vi "loopmod.vi"() -> ()   [LabVIEW 2018, in "sandbox.lvlib"]
uses:
  sandbox.lvlib
panel:
  in  "y":i32
  in  "x":i32
  out "floor(x/y)":i32
  out "x-y*floor(x/y)":i32
  in  "Stop Button":bool
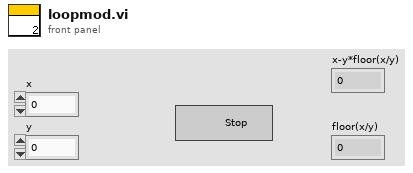
[diagram p1: front panel]
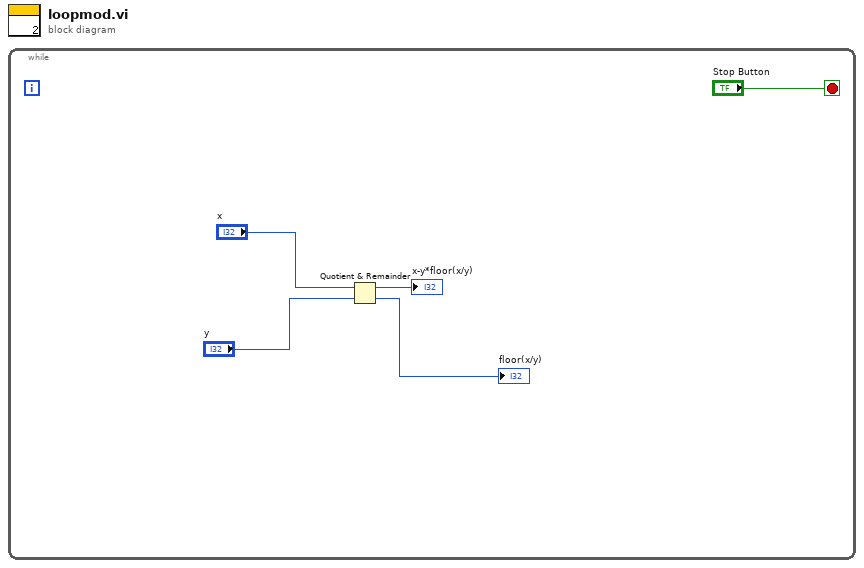
[diagram p0: block diagram]
diagram:
  n1 = while {
    stop <- "Stop Button" stop-if-true
    n2 = Quotient & Remainder(x="x", y="y") -> (x-y*floor(x/y)=→"x-y*floor(x/y)":i32, floor(x/y)=→"floor(x/y)":i32)
  }
